vi "GV FIFOOUT fpga enable.vi"() -> ()   [LabVIEW 2017]
panel:
  out "FIFOOUTfpgaEnable":bool
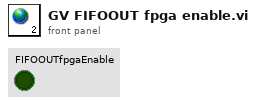
[diagram p1: front panel]
diagram:
